vi "CSM Example - State Machine Steps Executed on Sub-Module.vi"() -> ()   [LabVIEW 2017]
doc: "------------- lvcsm -------------\n[CSMStates]\nItem 0 = \"Event Structure\"\nItem 1 = \"Idle\"\nItem 2 = \"CSM Documentation\"\nItem 3 = \"VI Reference\"\nItem 4 = \"Error Handler\"\nItem 5 = \"Critical Error\"\nItem 6 = \"Target Timeout Error\"\nItem 7 = \"Target Error\"\nItem 8 = \"Async Response\"\nItem 9 = \"Response\"\nItem 10 = \"Async Message Posted\"\nItem 11 = \"Initialize Core Data\"\nItem 12 = \"Exit\"\nItem 13 = \"Data: Initialize\"\nItem 14 = \"Data: Cleanup\"\nItem 15 = \"Events: Register\"\nItem 16 = \"Events: Unregister\"\nItem 17 = \"UI: Initialize\"\nItem 18 = \"UI: Cursor Set\"\nItem 19 = \"UI: Front Panel State\"\nItem 20 = \"Macro: Initialize\"\nItem 21 = \"Macro: Exit\"\nItem 22 = \"Macro: SM\"\nItem 23 = \"SM: Step1\"\nItem 24 = \"SM: Step3\"\nItem 25 = \"SM: Event Check\"\n\n[CSMStatus]"
uses:
  user.lib/_NEVSTOP/Communicable State Machine(CSM)/Communicable State Machine.lvlib
panel:
  in  "Exit":bool
  in  "Run":bool
  out "State History of Sub-Module":string
  out "State History of Main":string
  # "SM: Step1\nSM: Step2 @ Sub-Module\nSM: Step3\nSM: Step4 @ Sub-Module\nSM: Event Check"
  # "(back to step1)"
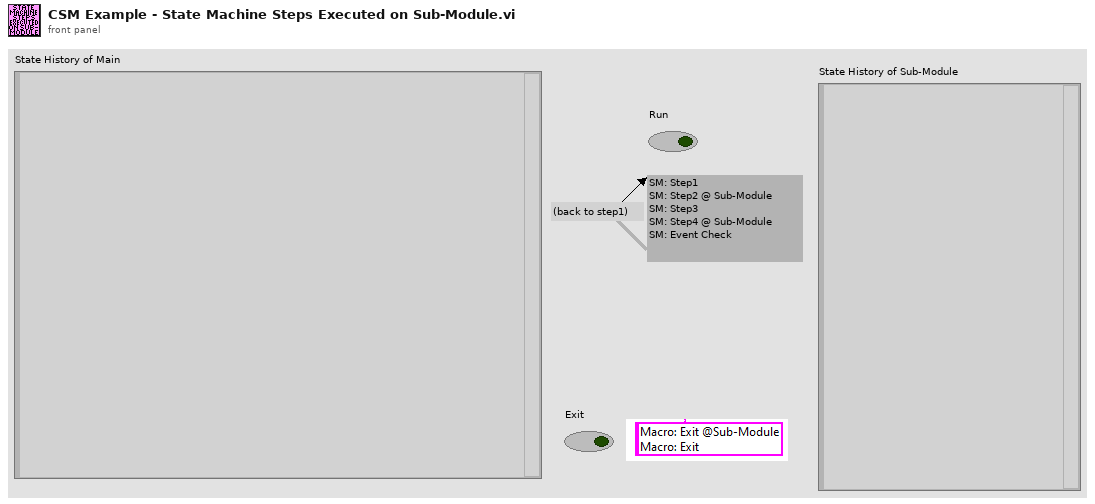
[diagram p1: front panel]
types:
  T1 = enum32{"Invalid", "Standard", "Closed", "Hidden", "Minimized", "Maximized"}
  T2 = enum32{"invalid app kind", "Development System", "Run Time System", "Student Edition", "Embedded LabVIEW", "Evaluation", "Custom"}
  T3 = typedef "Communicable State Machine.lvlib/_CSM_Response Source Message.ctl" = cluster{"‘State":string, "’Arguments":string, "’Error":errorcluster}
  T4 = cluster{"Current VI Reference":refnum<vi>, "Close Panel on Exit?":bool}
  T5 = cluster{"Core":cluster{"Current VI Reference":refnum<vi>, "Close Panel on Exit?":bool}, "Your Boolean data":bool, "State":string}
  T6 = cluster{"Core":cluster{"Current VI Reference":refnum<vi>, "Close Panel on Exit?":bool}, "Your Boolean data":bool, "Your string data":string}
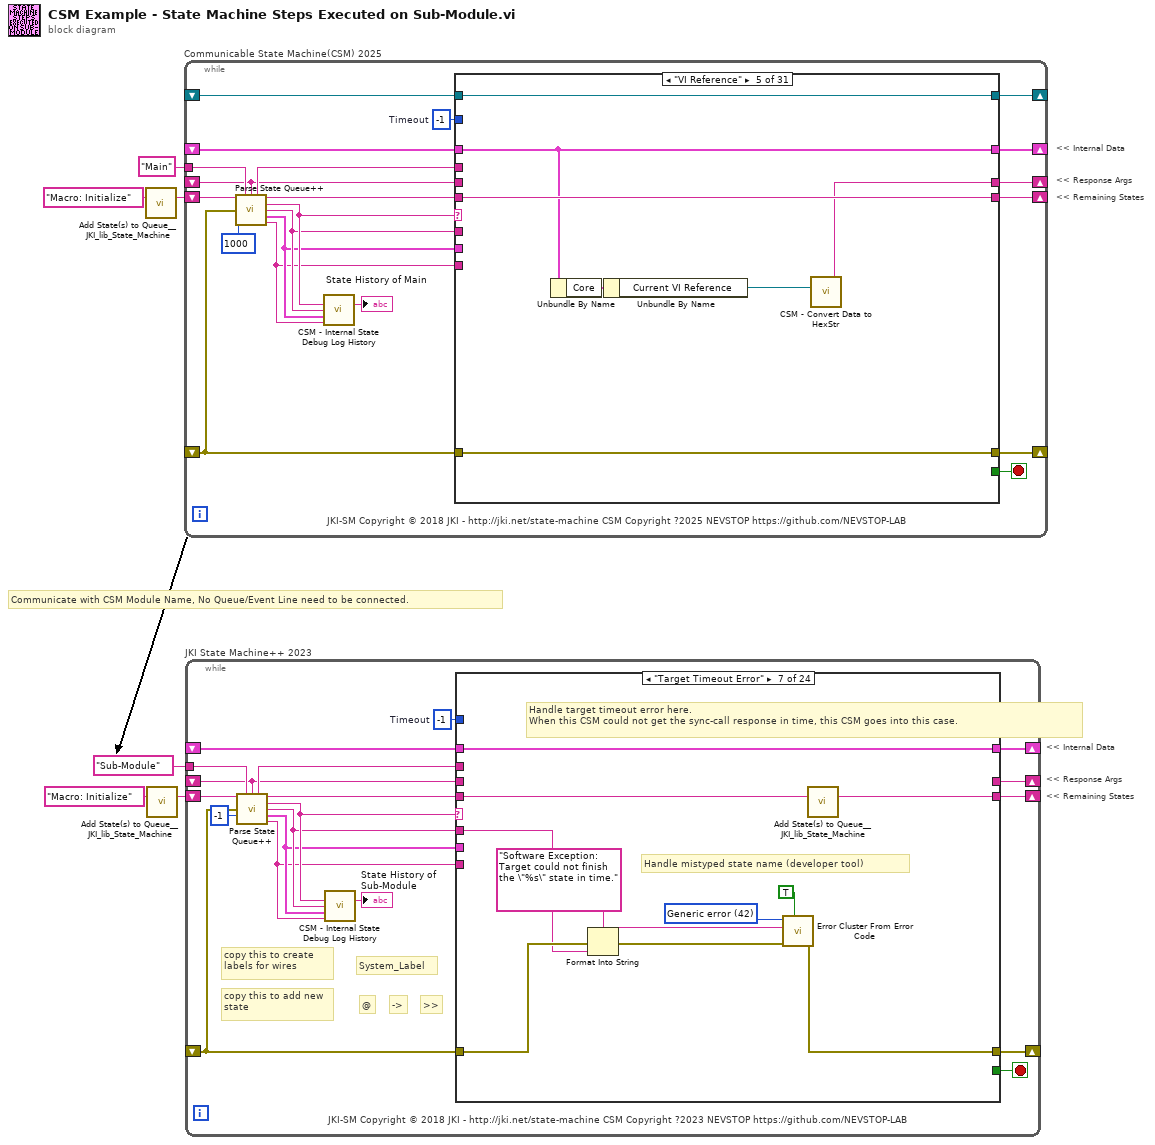
[diagram p0: block diagram]
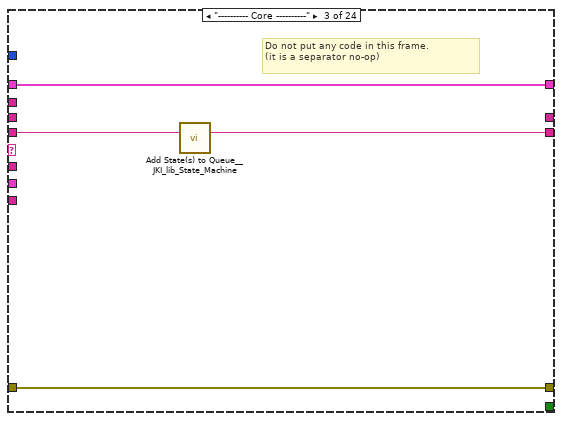
[diagram p4: hidden frame]
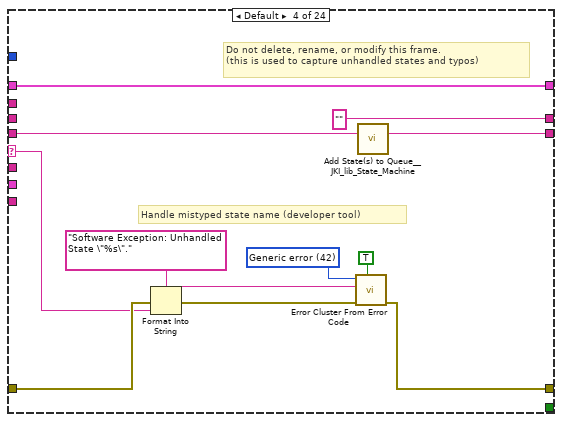
[diagram p5: hidden frame]
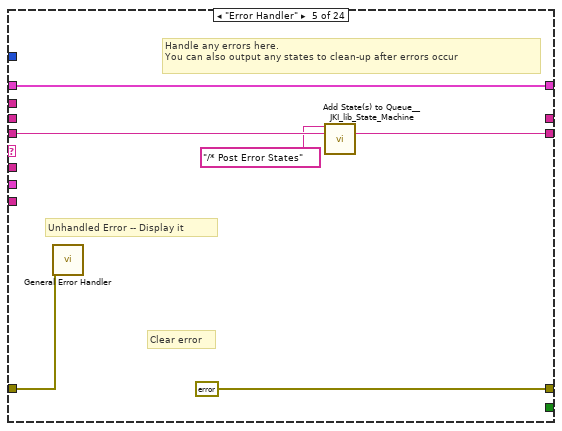
[diagram p6: hidden frame]
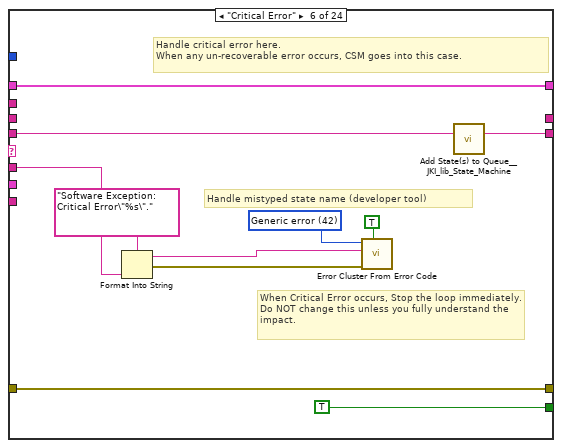
[diagram p7: hidden frame]
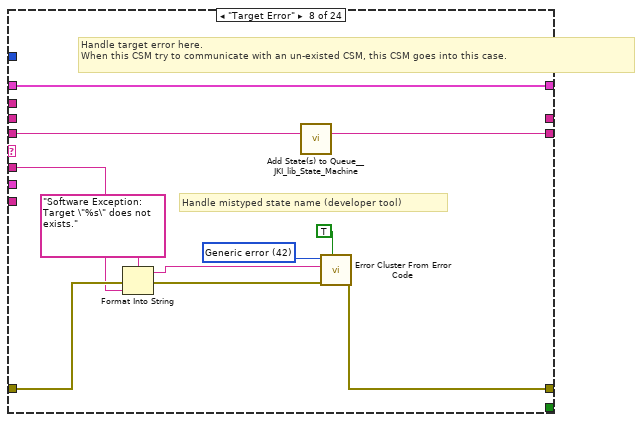
[diagram p8: hidden frame]
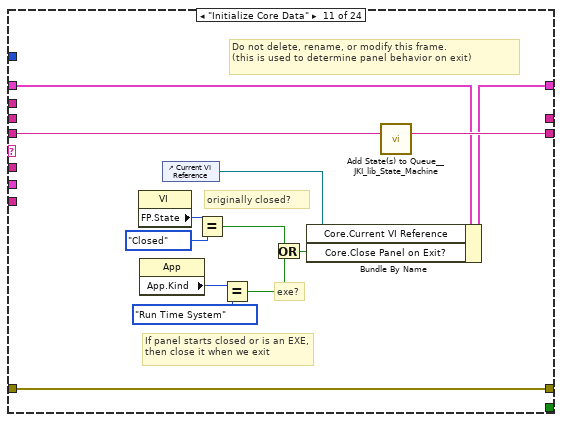
[diagram p11: hidden frame]
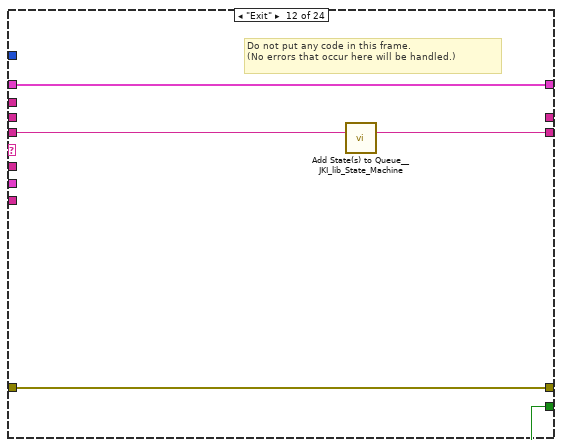
[diagram p12: hidden frame]
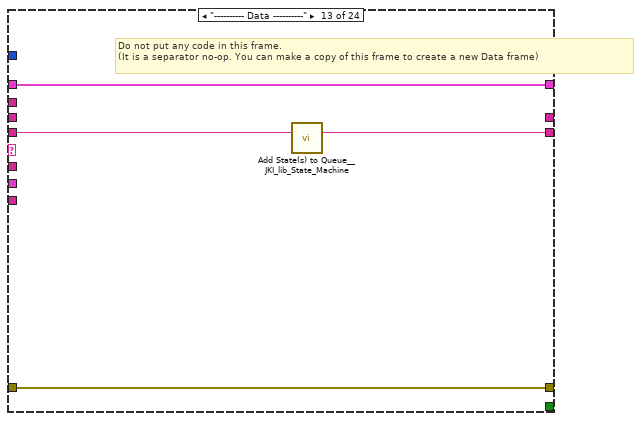
[diagram p13: hidden frame]
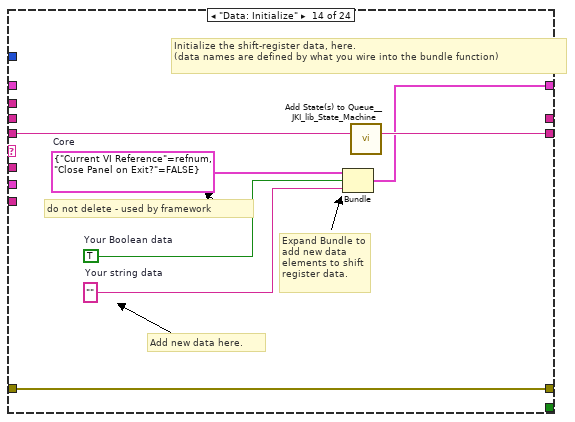
[diagram p14: hidden frame]
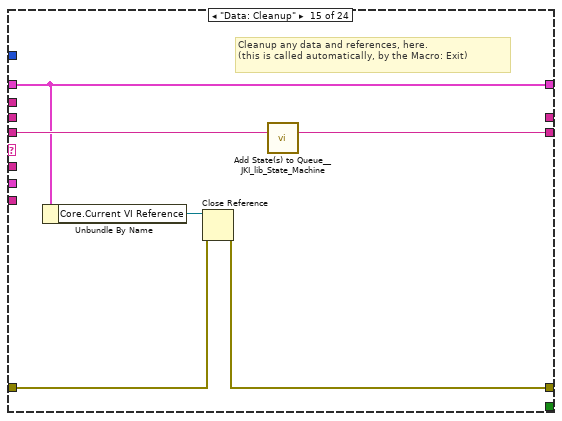
[diagram p15: hidden frame]
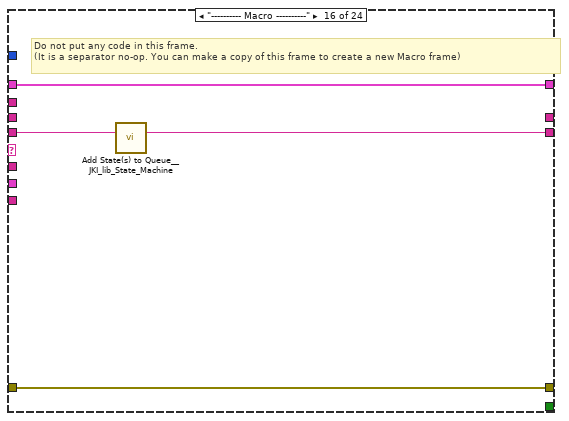
[diagram p16: hidden frame]
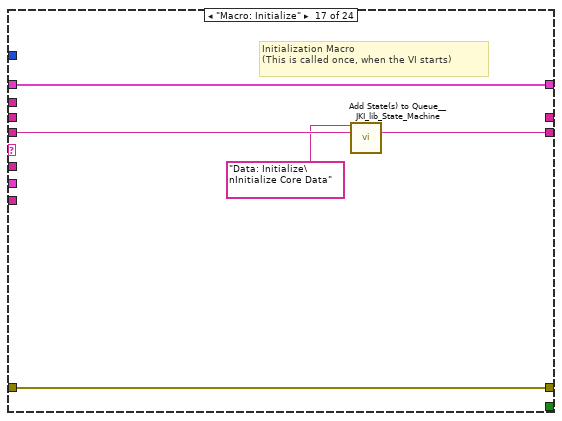
[diagram p17: hidden frame]
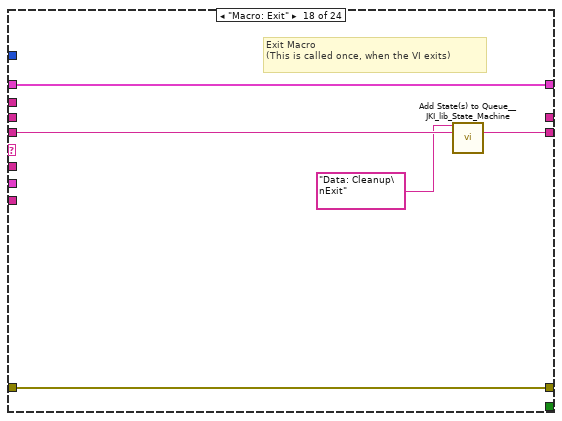
[diagram p18: hidden frame]
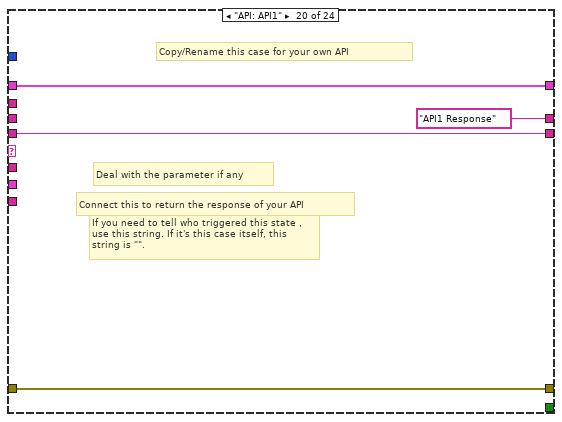
[diagram p20: hidden frame]
diagram:
  # "Communicate with CSM Module Name, No Queue/Event Line need to be connected."
  # "<< Internal Data"
  # "<< Response Args"
  # "<< Remaining States"
  # "<< Internal Data"
  # "<< Response Args"
  # "<< Remaining States"
  n1 = call <vilib>:"Add State(s) to Queue__JKI_lib_State_Machine.vi"("State(s) in (\"\")"="Macro: Initialize") -> ("States Out"=w6:string)  [unwired: 14 in]
  n2 = call <vilib>:"Add State(s) to Queue__JKI_lib_State_Machine.vi"("State(s) in (\"\")"="Macro: Initialize") -> ("States Out"=w1:string)  [unwired: 14 in]
  n3 = while "Communicable State Machine(CSM) 2025" {
    shift-right: [w8] -> _
    shift-left: _ -> [w22]
    shift-right: [w25] -> _
    shift-left: _ -> [w20]
    shift-right: [w24] -> _
    shift-left: w6 -> [w26]
    tunnel: "Main" ("Name(\"\" to use uuid)") -> [w15]
    shift-right: [w18] -> _
    shift-left: _ -> [w9]
    shift-right: [w17] -> _
    shift-left: _ -> [w16]
    stop <- w23 stop-if-true
    w21 = -1  # Timeout
    # "JKI-SM Copyright © 2018 JKI - http://jki.net/state-machine CSM Copyright ?2025 NEVSTOP https://github.com/NEVSTOP-LAB"
    n4 = call "Parse State Queue++.vi"("State Queue"=w26, "Name (\"\" to Use UUID)"=w15, "Response Arguments"=w9, "Previous Error"=w20, "Response Timeout (-2 Use Global Settings)"=1000 ("Response Timeout(1000ms)")) -> ("Name Used"=w10:string, "Remaining States"=w27:string, "Current State"=w14:string, "Arguments"=w13:string, ">> Response Source Message >>"=w12:T3, ">> Source CSM >>"=w11:string)  [unwired: 5 in]
    n5 = call "CSM - Internal State Debug Log History.vi"("State"=w14, "Arguments (\"\")"=w13, ">> Response Source Message >>"=w12, "Source (\"\")"=w11) -> ("Debug Log"=→"State History of Main":string)  [unwired: 11 in]
    n6 = case shown="\"VI Reference\"" w14 {
      selector: w14 -> [_ _ _ w72 _ _ _ _ _ _ _ _ _ _ _ _ _ _ _ _ _ _ _ _ _ _ _ _ _ _ _]
      tunnel: w27 -> [w30 w63 w69 w76 w88 w96 w106 w114 w126 w135 w139 w154 w160 w165 w173 w180 w185 w191 w195 w201 w207 w214 w226 w296 w302 w313 w316 w322 w328 w334 w342]
      tunnel: w13 -> [_ _ _ _ _ _ w99 w110 w122 _ _ _ _ _ _ _ _ _ _ _ _ w209 w220 _ _ _ _ _ _ _ _]
      tunnel: w22 -> [w35 w62 w66 w74 w87 w93 w107 w112 w124 w134 w138 w147 w158 w162 _ w175 w182 w190 w194 w198 w205 w212 w222 w293 w299 w310 w318 w321 w327 w333 w344]
      tunnel: [w34 w64 w67 w78 w89 errorcluster {"status"=FALSE, "code"=0, "source"=""} ("error out") w108 w116 w128 w136 w140 w151 w157 w163 w170 w176 w183 w186 w193 w199 w204 w210 w223 w294 w300 w311 w319 w323 w329 w335 w345] -> w25
      tunnel: w20 -> [w33 w64 w67 w77 w89 w92 w108 w115 w127 w136 w140 w151 w157 w163 w170 w177 w183 _ w196 w199 w204 w211 w224 w294 w300 w311 w319 w323 w329 w335 w345]
      tunnel: [w36 w63 w68 w75 w88 w95 w105 w113 w125 w135 w139 w153 w159 w164 w172 w179 w184 w191 w195 w200 w206 w213 w225 w295 w301 w312 w315 w322 w328 w334 w341] -> w24
      tunnel: [_ _ _ _ _ _ TRUE _ _ _ _ _ TRUE _ _ _ _ _ _ _ _ _ _ _ _ _ _ _ _ _ _] -> w23
      tunnel: [w32 w62 w66 w74 w87 w93 w107 w112 w124 w134 w138 w152 w158 w162 w171 w175 w182 w190 w194 w198 w205 w212 w222 w293 w299 w310 w318 w321 w327 w333 w344] -> w8
      tunnel: w21 -> [w29 _ _ _ _ _ _ _ _ _ _ _ _ _ _ _ _ _ _ _ _ _ _ _ _ _ _ _ _ _ _]
      tunnel: w11 -> [_ _ _ _ _ _ _ _ _ _ _ _ _ _ _ _ _ _ _ _ _ _ _ _ _ _ _ _ _ _ _]
      tunnel: w12 -> [_ _ _ _ _ _ _ _ _ _ _ _ _ _ _ _ _ _ _ _ _ _ _ _ _ _ _ _ _ _ _]
      tunnel: [_ _ _ "" w83 _ _ _ _ _ _ _ _ _ _ _ _ _ _ _ _ _ _ _ _ _ _ _ "Step1 Finished" "Step3 Finished" _] -> w18
      tunnel: [w31 w61 w65 w70 w86 w90 w97 w109 w121 w133 w137 w141 w155 w161 w166 w174 w181 w189 w192 w197 w203 w208 w219 w292 w297 w303 w317 w320 w326 w332 w343] -> w17
      tunnel: w16 -> [w31 w61 w65 w70 w86 w90 w97 w109 w121 w133 w137 w141 w155 w161 w166 w174 w181 _ w192 w197 w203 w208 w219 w292 w297 w303 w317 w320 w326 w332 w343]
      tunnel: w10 -> [_ _ _ _ _ _ _ _ _ _ _ _ _ _ _ _ _ w188 _ _ _ _ _ _ _ _ _ _ _ _ _]
      tunnel: w9 -> [_ _ _ _ _ _ _ _ _ _ _ _ _ _ _ _ _ _ _ _ _ _ _ _ _ _ _ _ _ _ _]
      frame "", "Event Structure", "Idle" {
        # "executes when the state queue is empty"
        n7 = call "Timeout Selector.vi"("Remaining States"=w30, "Timeout Expected"=w29) -> ("Timeout"=w28:i32)  [unwired: 5 in]
        n8 = event shown="[2] \"Run\": Value Change" {
          selector: w31 -> [_ _ _ _ _]
          dyn-events: _ -> [_ _ _ _ _]
          timeout: w28 -> [_ _ _ _ _]
          tunnel: w30 -> [w40 w42 w46 w55 w60]
          tunnel: [w39 w42 w47 w54 w59] -> w36
          tunnel: w35 -> [w37 w43 w48 w52 w57]
          tunnel: [w38 w41 w49 w53 w58] -> w34
          tunnel: w33 -> [w38 w41 w49 w53 w58]
          tunnel: [w37 w43 w48 w52 w57] -> w32
          event Timeout {
            n9 = event-data() -> ()  [unwired: 1 in, 1 out]
            n10 = call <vilib>:"Add State(s) to Queue__JKI_lib_State_Machine.vi"("State(s) in (\"\")"=w40) -> ("States Out"=w39:string)  [unwired: 14 in]
          }
          event User Event {
            # "This user event is used to break out CSM from waiting in the event structure, to process the next state from external. DO NOT place any code here unless you really need to."
            n11 = event-data() -> ()  [unwired: 1 in, 1 out]
          }
          event "Run": Value Change {
            n12 = event-data() -> ("NewVal"=w45:bool)  [unwired: 1 in]
            n13 = call "Add State(s) to Queue By BOOL(Element).vi"("TRUE (\"\")"="Macro: SM" ("TRUE(Empty)"), "Condition"=w45, "State Queue (\"\")"=w46) -> ("Remaining States"=w47:string)  [unwired: 8 in]
          }
          event Panel Close? {
            # "Discard the event because we'll close the front panel ourselves in Macro: Exit"
            # "Close Panel button (pressed) Event\n(this executes Macro: Exit to terminate the VI)"
            n14 = event-data() -> ()  [unwired: 1 in, 1 out]
            n15 = call <vilib>:"Add State(s) to Queue__JKI_lib_State_Machine.vi"("State(s) in Front (\"\")"="Macro: Exit @ Message Handler\nMacro: Exit", "State(s) in (\"\")"=w55) -> ("States Out"=w54:string)  [unwired: 13 in]
            n16 = event-data("Discard?"=TRUE) -> ()  [unwired: 1 in, 1 out]
          }
          event "Exit": Value Change {
            # "Close Panel button (pressed) Event\n(this executes Macro: Exit to terminate the VI)"
            n17 = event-data() -> ()  [unwired: 1 in, 6 out]
            n18 = call <vilib>:"Add State(s) to Queue__JKI_lib_State_Machine.vi"("State(s) in Front (\"\")"="Macro: Exit -@Sub-Module\nMacro: Exit", "State(s) in (\"\")"=w60) -> ("States Out"=w59:string)  [unwired: 13 in]
          }
        }
      }
      frame "CSM Documentation" {
        # "Commenting:\nTo add a comment use \"//\" or \"#\" and all text to the right will be ignored\nCommenting Example:\nUI: Initialize // This initializes the UI\n# This whole line is a comment\n// Another comment line"
        # "State Syntax:\nStateCategory: State >> Argument @ CSMName\nStateCategory: State >> Argument -> CSMName\n\nLine Terminator: Line feed"
        # "CSM Documentation"
      }
      frame "---------- Core ----------" {
        # "Do not put any code in this frame.\n(it is a separator no-op)"
        n19 = call <vilib>:"Add State(s) to Queue__JKI_lib_State_Machine.vi"("State(s) in (\"\")"=w69) -> ("States Out"=w68:string)  [unwired: 14 in]
      }
      frame Default {
        w81 = 42 items=["No error", "Argument error", "Memory is full", "Out of zone", "End of file", "File already open", "Generic file I/O error", "File not found", "File permission error", "Disk is full", "Duplicate path", "Too many files open", "System feature not enabled", "Resource file not found", "Cannot add resource", "Resource not found", "Image not found", "Image memory error", "Pen does not exist", "Config type invalid", "Config token not found", "Config parse error", "Config memory error", "Bad external code format", "Bad external code offset", "External code not present", "Null window", "Destroy window error", "Null menu", "Print aborted", "Bad print record", "Print driver error", "Windows error during printing", "Memory error during printing", "Print dialog error", "Generic print error", "Invalid device refnum", "Device not found", "Device parameter error", "Device unit error", "Cannot open device", "Device call aborted", "Generic error", "Cancelled by user", "Object ID too low", "Object ID too high", "Object not in heap", "Unknown heap", "Unknown object (invalid DefProc)", "Unknown object (DefProc not in table)", "Message out of range", "Invalid (null) method", "Unknown message", "Manager call not supported", "Bad address", "Network operation in progress", "Network operation timed out", "Connection is busy", "Network attribute not supported", "Network error", "Address in use", "System out of memory", "Connection aborted", "Connection refused", "Not connected", "Already connected", "Connection closed", "Initialization error (interapplication manager)", "Bad occurrence", "Wait on unbound occurrence handler", "Occurrence queue overflow", "Datalog type conflict", "Unused", "Unrecognized type (interapplication manager)", "Memory corrupt", "Failed to make temporary DLL", "Old CIN version", "Drag socket not found", "Failed to load drop-object", "Failed to register OLE object", "Failed to release OLE object", "Format specifier type mismatch", "Unknown format specifier", "Too few format specifiers", "Too many format specifiers", "Scan failed", "Newer CIN version", "Error converting to variant", "Runtime menu error", "Password tampered", "Variant attribute not found", "Incompatible variant data type", "Event data is not available", "Event Store is not present", "Occurrence is not found", "Event Queue is not created", "Event info is not available", "Refnum passed is NULL", "Error retrieving Class GUID", "Error retrieving CoClass GUID", "Error retrieving TypeLib GUID.", "Bad built application magic bytes.", "Specific driver is different from the specific driver associated with the Logical Name.", "There is no session opened to the class driver.", "Max Error", "MAX - Error with config objects", "MAX - Error loading configuration", "MAX - Group not supported"]
        # "Do not delete, rename, or modify this frame.\n(this is used to capture unhandled states and typos)"
        # "Handle mistyped state name (developer tool)"
        n20 = Format Into String(format string="Software Exception: Unhandled State \"%s\"." ("message"), error in=w77, w72) -> (resulting string=w80:string, error out=w79:errorcluster)  [unwired: 1 in]
        n21 = call <vilib>:"Error Cluster From Error Code.vi"("show call chain? (False)"=TRUE, "error in (no error)"=w79, "error message (\"\")"=w80, "error code (0)"=w81) -> ("error out"=w78:errorcluster)  [unwired: 5 in]
        n22 = call <vilib>:"Add State(s) to Queue__JKI_lib_State_Machine.vi"("State(s) in (\"\")"=w76) -> ("States Out"=w75:string)  [unwired: 14 in]
      }
      frame "VI Reference" {
        n23 = Unbundle By Name(w87) -> ("Core"=w85:T4)
        n24 = Unbundle By Name(w85) -> ("Current VI Reference"=w84:refnum<vi>)
        n25 = call "CSM - Convert Data to HexStr.vi"("Variant"=w84) -> ("HEX String (0-9,A-F)"=w83:string)  [unwired: 8 in]
      }
      frame "Error Handler" {
        # "Unhandled Error -- Display it"
        # "Handle any errors here.\nYou can also output any states to clean-up after errors occur"
        # "Clear error"
        n26 = call <vilib>:"General Error Handler.vi"("error in (no error)"=w92) -> ()  [unwired: 10 in, 5 out]
        n27 = call <vilib>:"Add State(s) to Queue__JKI_lib_State_Machine.vi"("State(s) in Front (\"\")"="/* Post Error States", "State(s) in (\"\")"=w96) -> ("States Out"=w95:string)  [unwired: 13 in]
      }
      frame "Critical Error" {
        w103 = 42 items=["No error", "Argument error", "Memory is full", "Out of zone", "End of file", "File already open", "Generic file I/O error", "File not found", "File permission error", "Disk is full", "Duplicate path", "Too many files open", "System feature not enabled", "Resource file not found", "Cannot add resource", "Resource not found", "Image not found", "Image memory error", "Pen does not exist", "Config type invalid", "Config token not found", "Config parse error", "Config memory error", "Bad external code format", "Bad external code offset", "External code not present", "Null window", "Destroy window error", "Null menu", "Print aborted", "Bad print record", "Print driver error", "Windows error during printing", "Memory error during printing", "Print dialog error", "Generic print error", "Invalid device refnum", "Device not found", "Device parameter error", "Device unit error", "Cannot open device", "Device call aborted", "Generic error", "Cancelled by user", "Object ID too low", "Object ID too high", "Object not in heap", "Unknown heap", "Unknown object (invalid DefProc)", "Unknown object (DefProc not in table)", "Message out of range", "Invalid (null) method", "Unknown message", "Manager call not supported", "Bad address", "Network operation in progress", "Network operation timed out", "Connection is busy", "Network attribute not supported", "Network error", "Address in use", "System out of memory", "Connection aborted", "Connection refused", "Not connected", "Already connected", "Connection closed", "Initialization error (interapplication manager)", "Bad occurrence", "Wait on unbound occurrence handler", "Occurrence queue overflow", "Datalog type conflict", "Unused", "Unrecognized type (interapplication manager)", "Memory corrupt", "Failed to make temporary DLL", "Old CIN version", "Drag socket not found", "Failed to load drop-object", "Failed to register OLE object", "Failed to release OLE object", "Format specifier type mismatch", "Unknown format specifier", "Too few format specifiers", "Too many format specifiers", "Scan failed", "Newer CIN version", "Error converting to variant", "Runtime menu error", "Password tampered", "Variant attribute not found", "Incompatible variant data type", "Event data is not available", "Event Store is not present", "Occurrence is not found", "Event Queue is not created", "Event info is not available", "Refnum passed is NULL", "Error retrieving Class GUID", "Error retrieving CoClass GUID", "Error retrieving TypeLib GUID.", "Bad built application magic bytes.", "Specific driver is different from the specific driver associated with the Logical Name.", "There is no session opened to the class driver.", "Max Error", "MAX - Error with config objects", "MAX - Error loading configuration", "MAX - Group not supported"]
        # "Handle critical error here.\nWhen any un-recoverable error occurs, CSM goes into this case."
        # "When Critical Error occurs, Stop the loop immediately. Do NOT change this unless you fully understand the impact."
        # "Handle mistyped state name (developer tool)"
        n28 = Format Into String(format string="Software Exception: Critical Error\"%s\"." ("message"), w99) -> (resulting string=w102:string, error out=w101:errorcluster)  [unwired: 2 in]
        n29 = call <vilib>:"Error Cluster From Error Code.vi"("show call chain? (False)"=TRUE, "error in (no error)"=w101, "error message (\"\")"=w102, "error code (0)"=w103) -> ()  [unwired: 5 in, 1 out]
        n30 = call <vilib>:"Add State(s) to Queue__JKI_lib_State_Machine.vi"("State(s) in (\"\")"=w106) -> ("States Out"=w105:string)  [unwired: 14 in]
      }
      frame "Target Timeout Error" {
        w119 = 42 items=["No error", "Argument error", "Memory is full", "Out of zone", "End of file", "File already open", "Generic file I/O error", "File not found", "File permission error", "Disk is full", "Duplicate path", "Too many files open", "System feature not enabled", "Resource file not found", "Cannot add resource", "Resource not found", "Image not found", "Image memory error", "Pen does not exist", "Config type invalid", "Config token not found", "Config parse error", "Config memory error", "Bad external code format", "Bad external code offset", "External code not present", "Null window", "Destroy window error", "Null menu", "Print aborted", "Bad print record", "Print driver error", "Windows error during printing", "Memory error during printing", "Print dialog error", "Generic print error", "Invalid device refnum", "Device not found", "Device parameter error", "Device unit error", "Cannot open device", "Device call aborted", "Generic error", "Cancelled by user", "Object ID too low", "Object ID too high", "Object not in heap", "Unknown heap", "Unknown object (invalid DefProc)", "Unknown object (DefProc not in table)", "Message out of range", "Invalid (null) method", "Unknown message", "Manager call not supported", "Bad address", "Network operation in progress", "Network operation timed out", "Connection is busy", "Network attribute not supported", "Network error", "Address in use", "System out of memory", "Connection aborted", "Connection refused", "Not connected", "Already connected", "Connection closed", "Initialization error (interapplication manager)", "Bad occurrence", "Wait on unbound occurrence handler", "Occurrence queue overflow", "Datalog type conflict", "Unused", "Unrecognized type (interapplication manager)", "Memory corrupt", "Failed to make temporary DLL", "Old CIN version", "Drag socket not found", "Failed to load drop-object", "Failed to register OLE object", "Failed to release OLE object", "Format specifier type mismatch", "Unknown format specifier", "Too few format specifiers", "Too many format specifiers", "Scan failed", "Newer CIN version", "Error converting to variant", "Runtime menu error", "Password tampered", "Variant attribute not found", "Incompatible variant data type", "Event data is not available", "Event Store is not present", "Occurrence is not found", "Event Queue is not created", "Event info is not available", "Refnum passed is NULL", "Error retrieving Class GUID", "Error retrieving CoClass GUID", "Error retrieving TypeLib GUID.", "Bad built application magic bytes.", "Specific driver is different from the specific driver associated with the Logical Name.", "There is no session opened to the class driver.", "Max Error", "MAX - Error with config objects", "MAX - Error loading configuration", "MAX - Group not supported"]
        # "Handle target timeout error here.\nWhen this CSM could not get the sync-call response in time, this CSM goes into this case."
        # "Handle mistyped state name (developer tool)"
        n31 = Format Into String(format string="Software Exception: Target could not finish the \"%s\" state in time." ("message"), error in=w115, w110) -> (resulting string=w118:string, error out=w117:errorcluster)  [unwired: 1 in]
        n32 = call <vilib>:"Error Cluster From Error Code.vi"("show call chain? (False)"=TRUE, "error in (no error)"=w117, "error message (\"\")"=w118, "error code (0)"=w119) -> ("error out"=w116:errorcluster)  [unwired: 5 in]
        n33 = call <vilib>:"Add State(s) to Queue__JKI_lib_State_Machine.vi"("State(s) in (\"\")"=w114) -> ("States Out"=w113:string)  [unwired: 14 in]
      }
      frame "Target Error" {
        w131 = 42 items=["No error", "Argument error", "Memory is full", "Out of zone", "End of file", "File already open", "Generic file I/O error", "File not found", "File permission error", "Disk is full", "Duplicate path", "Too many files open", "System feature not enabled", "Resource file not found", "Cannot add resource", "Resource not found", "Image not found", "Image memory error", "Pen does not exist", "Config type invalid", "Config token not found", "Config parse error", "Config memory error", "Bad external code format", "Bad external code offset", "External code not present", "Null window", "Destroy window error", "Null menu", "Print aborted", "Bad print record", "Print driver error", "Windows error during printing", "Memory error during printing", "Print dialog error", "Generic print error", "Invalid device refnum", "Device not found", "Device parameter error", "Device unit error", "Cannot open device", "Device call aborted", "Generic error", "Cancelled by user", "Object ID too low", "Object ID too high", "Object not in heap", "Unknown heap", "Unknown object (invalid DefProc)", "Unknown object (DefProc not in table)", "Message out of range", "Invalid (null) method", "Unknown message", "Manager call not supported", "Bad address", "Network operation in progress", "Network operation timed out", "Connection is busy", "Network attribute not supported", "Network error", "Address in use", "System out of memory", "Connection aborted", "Connection refused", "Not connected", "Already connected", "Connection closed", "Initialization error (interapplication manager)", "Bad occurrence", "Wait on unbound occurrence handler", "Occurrence queue overflow", "Datalog type conflict", "Unused", "Unrecognized type (interapplication manager)", "Memory corrupt", "Failed to make temporary DLL", "Old CIN version", "Drag socket not found", "Failed to load drop-object", "Failed to register OLE object", "Failed to release OLE object", "Format specifier type mismatch", "Unknown format specifier", "Too few format specifiers", "Too many format specifiers", "Scan failed", "Newer CIN version", "Error converting to variant", "Runtime menu error", "Password tampered", "Variant attribute not found", "Incompatible variant data type", "Event data is not available", "Event Store is not present", "Occurrence is not found", "Event Queue is not created", "Event info is not available", "Refnum passed is NULL", "Error retrieving Class GUID", "Error retrieving CoClass GUID", "Error retrieving TypeLib GUID.", "Bad built application magic bytes.", "Specific driver is different from the specific driver associated with the Logical Name.", "There is no session opened to the class driver.", "Max Error", "MAX - Error with config objects", "MAX - Error loading configuration", "MAX - Group not supported"]
        # "Handle target error here.\nWhen this CSM try to communicate with an un-existed CSM, this CSM goes into this case."
        # "Handle mistyped state name (developer tool)"
        n34 = Format Into String(format string="Software Exception: Target \"%s\" does not exists." ("message"), error in=w127, w122) -> (resulting string=w130:string, error out=w129:errorcluster)  [unwired: 1 in]
        n35 = call <vilib>:"Add State(s) to Queue__JKI_lib_State_Machine.vi"("State(s) in (\"\")"=w126) -> ("States Out"=w125:string)  [unwired: 14 in]
        n36 = call <vilib>:"Error Cluster From Error Code.vi"("show call chain? (False)"=TRUE, "error in (no error)"=w129, "error message (\"\")"=w130, "error code (0)"=w131) -> ("error out"=w128:errorcluster)  [unwired: 5 in]
      }
      frame "Async Response", "Response" {
        # "Handle Async-call Response (\"Async Response\" for ->)"
        # "Handle Sync-call Response (\"Response\" for @)"
        # "After Message is executed, CSM goes to this state for receive the response. \n    For Async Message(->), \"Async Response\" is used. This CSM will goes to \"Async Message Posted\" immediately and receive the \"Async Response\" after the callee finishes the message.\n    For Sync Message(@),  This CSM will wait until the message is done and immediately goes to \"Response\""
      }
      frame "Async Message Posted" {
        # "Handle post action for async message (->)."
        # "After Async Message is posted (->), CSM goes to this state for post-action. You can use Argument - State to tell which Async Message is called."
      }
      frame "Initialize Core Data" {
        # "Do not delete, rename, or modify this frame.\n(this is used to determine panel behavior on exit)"
        # "originally closed?"
        # "exe?"
        # "If panel starts closed or is an EXE, then close it when we exit"
        n37 = property class="VI"() -> ("FP.State"=w144:T1)  [unwired: 2 in, 2 out]
        n38 = property class="App"() -> ("App.Kind"=w150:T2)  [unwired: 2 in, 2 out]
        n39 = control-ref of="Current VI Reference"() -> (w145:refnum<vi>)
        n40 = Equal?(x=w144, y=T1."Closed" ("Front Panel Window:State")) -> (x = y?=w142:bool)
        n41 = Equal?(x=w150, y=T2."Run Time System" ("Application:Kind")) -> (x = y?=w148:bool)
        n42 = Or(x=w142, y=w148) -> (x .or. y?=w146:bool)
        n43 = Bundle By Name(cluster=w147, "Core.Current VI Reference"=w145, "Core.Close Panel on Exit?"=w146) -> (w152:T5)
        n44 = call <vilib>:"Add State(s) to Queue__JKI_lib_State_Machine.vi"("State(s) in (\"\")"=w154) -> ("States Out"=w153:string)  [unwired: 14 in]
      }
      frame "Exit" {
        # "Do not put any code in this frame.\n(No errors that occur here will be handled.)"
        n45 = call <vilib>:"Add State(s) to Queue__JKI_lib_State_Machine.vi"("State(s) in (\"\")"=w160) -> ("States Out"=w159:string)  [unwired: 14 in]
      }
      frame "---------- Data ----------" {
        # "Do not put any code in this frame.\n(It is a separator no-op. You can make a copy of this frame to create a new Data frame)"
        n46 = call <vilib>:"Add State(s) to Queue__JKI_lib_State_Machine.vi"("State(s) in (\"\")"=w165) -> ("States Out"=w164:string)  [unwired: 14 in]
      }
      frame "Data: Initialize" {
        w167 = T4 {"Current VI Reference"=refnum, "Close Panel on Exit?"=FALSE}  # Core
        w169 = TRUE  # Your Boolean data
        w168 = ""  # State
        # "do not delete - used by framework"
        # "Initialize the shift-register data, here.\n(data names are defined by what you wire into the bundle function)"
        n47 = Bundle("Core"=w167, "Your Boolean data"=w169, "State"=w168) -> (w171:T5)  [unwired: 1 in]
        n48 = call <vilib>:"Add State(s) to Queue__JKI_lib_State_Machine.vi"("State(s) in (\"\")"=w173) -> ("States Out"=w172:string)  [unwired: 14 in]
      }
      frame "Data: Cleanup" {
        # "Cleanup any data and references, here.\n(this is called automatically, by the Macro: Exit)"
        n49 = Unbundle By Name(w175) -> ("Core.Current VI Reference"=w178:refnum<vi>)
        n50 = Close Reference(reference=w178, error in (no error)=w177) -> (error out=w176:errorcluster)
        n51 = call <vilib>:"Add State(s) to Queue__JKI_lib_State_Machine.vi"("State(s) in (\"\")"=w180) -> ("States Out"=w179:string)  [unwired: 14 in]
      }
      frame "---------- Events ----------" {
        # "Do not put any code in this frame.\n(It is a separator no-op. You can make a copy of this frame to create a new UI frame)"
        n52 = call <vilib>:"Add State(s) to Queue__JKI_lib_State_Machine.vi"("State(s) in (\"\")"=w185) -> ("States Out"=w184:string)  [unwired: 14 in]
      }
      frame "Events: Register" {
        # "Register message event to break Waiting in Event structure."
        n53 = call "CSM - Get New State Notifier Event.vi"("Name (\"\" to Use UUID) In"=w188) -> ("error out"=w186:errorcluster, "New State Notifier Event"=w187:refnum<user-event>)  [unwired: 9 in]
        n54 = register-events(w187) -> (reference out=w189:refnum<event-registration>)  [unwired: 2 in, 1 out]
      }
      frame "Events: Unregister" {
        n55 = Unregister For Events(event registration refnum=w192, error in=w196) -> (error out=w193:errorcluster)
      }
      frame "---------- UI ----------" {
        # "Do not put any code in this frame.\n(It is a separator no-op. You can make a copy of this frame to create a new UI frame)"
        n56 = call <vilib>:"Add State(s) to Queue__JKI_lib_State_Machine.vi"("State(s) in (\"\")"=w201) -> ("States Out"=w200:string)  [unwired: 14 in]
      }
      frame "UI: Initialize" {
        # "Initialize the User Interface, here.\n(this is called automatically, by the Macro: Init)"
        n57 = local write "Run"(FALSE ("Run")) -> ()
        n58 = call <vilib>:"Add State(s) to Queue__JKI_lib_State_Machine.vi"("State(s) in (\"\")"=w207) -> ("States Out"=w206:string)  [unwired: 14 in]
      }
      frame "UI: Cursor Set" {
        # "Argument"
        # "Set and Unset Cursor Busy.\n(Usage: \"UI: Cursor Set >> Busy|Idle\")"
        n59 = case shown="\"Idle\", Default" w209 {
          tunnel: w211 -> [w216 w218]
          tunnel: [w215 w217] -> w210
          frame "Idle", Default {
            n60 = call <vilib>:"Unset Busy.vi"("error in (no error)"=w216) -> ("error out"=w215:errorcluster)  [unwired: 10 in]
          }
          frame "Busy" {
            n61 = call <vilib>:"Set Busy.vi"("error in (no error)"=w218) -> ("error out"=w217:errorcluster)  [unwired: 9 in, 1 out]
          }
        }
        n62 = call <vilib>:"Add State(s) to Queue__JKI_lib_State_Machine.vi"("State(s) in (\"\")"=w214) -> ("States Out"=w213:string)  [unwired: 14 in]
      }
      frame "UI: Front Panel State" {
        # "Argument"
        # "Set Front Panel Open or Closed\n(Usage: \"UI: Front Panel State >> Open|Close\")"
        n63 = Unbundle By Name(w222) -> ("Core.Current VI Reference"=w221:refnum<vi>)
        n64 = call <vilib>:"Add State(s) to Queue__JKI_lib_State_Machine.vi"("State(s) in (\"\")"=w226) -> ("States Out"=w225:string)  [unwired: 14 in]
        n65 = case shown="\"Minimize\", \"Minimized\"" w220 {
          tunnel: w224 -> [w232 w247 w258 w271 w284]
          tunnel: [w234 w248 w260 w273 w286] -> w223
          tunnel: w221 -> [w233 w245 w259 w272 w285]
          frame "Open", "Standard", Default {
            w227 = T1."Standard" ("State")
            n66 = property class="VI"(reference=w233, error in=w232) -> (reference out=w230:refnum<vi>, error out=w231:errorcluster, "FP.State"=w229:T1)
            n67 = Not Equal?(x=w229, y=w227) -> (x != y?=w228:bool)
            n68 = case shown="True" w228 {
              tunnel: [w238 w240] -> w234
              tunnel: w231 -> [w237 w240]
              tunnel: w230 -> [w236 _]
              tunnel: w227 -> [w235 _]
              frame True {
                n69 = invoke class="VI" method="FP.Open"(reference=w236, error in=w237, "Activate"=TRUE, "State"=w235) -> (error out=w238:errorcluster)  [unwired: 1 in, 4 out]
              }
              frame False {
              }
            }
          }
          frame "Close", "Closed" {
            n70 = property class="VI"(reference=w245, error in=w247) -> (reference out=w244:refnum<vi>, error out=w246:errorcluster, "FP.State"=w242:T1)
            n71 = Not Equal?(x=w242, y=T1."Closed" ("Front Panel Window:State")) -> (x != y?=w241:bool)
            n72 = case shown="True" w241 {
              tunnel: [w249 w252] -> w248
              tunnel: w246 -> [w249 w251]
              tunnel: w244 -> [_ w250]
              frame False {
              }
              frame True {
                n73 = invoke class="VI" method="FP.Close"(reference=w250, error in=w251) -> (error out=w252:errorcluster)  [unwired: 1 in, 2 out]
              }
            }
          }
          frame "Hidden", "Hide" {
            w253 = T1."Hidden" ("State")
            n74 = property class="VI"(reference=w259, error in=w258) -> (reference out=w256:refnum<vi>, error out=w257:errorcluster, "FP.State"=w255:T1)
            n75 = Not Equal?(x=w255, y=w253) -> (x != y?=w254:bool)
            n76 = case shown="True" w254 {
              tunnel: [w264 w265] -> w260
              tunnel: w257 -> [w263 w265]
              tunnel: w256 -> [w262 _]
              tunnel: w253 -> [w261 _]
              frame True {
                n77 = invoke class="VI" method="FP.Open"(reference=w262, error in=w263, "State"=w261) -> (error out=w264:errorcluster)  [unwired: 2 in, 4 out]
              }
              frame False {
              }
            }
          }
          frame "Minimize", "Minimized" {
            w266 = T1."Minimized" ("State")
            n78 = property class="VI"(reference=w272, error in=w271) -> (reference out=w269:refnum<vi>, error out=w270:errorcluster, "FP.State"=w268:T1)
            n79 = Not Equal?(x=w268, y=w266) -> (x != y?=w267:bool)
            n80 = case shown="True" w267 {
              tunnel: [w277 w278] -> w273
              tunnel: w270 -> [w276 w278]
              tunnel: w269 -> [w275 _]
              tunnel: w266 -> [w274 _]
              frame True {
                n81 = invoke class="VI" method="FP.Open"(reference=w275, error in=w276, "State"=w274) -> (error out=w277:errorcluster)  [unwired: 2 in, 4 out]
              }
              frame False {
              }
            }
          }
          frame "Maximize", "Maximized" {
            w279 = T1."Maximized" ("State")
            n82 = property class="VI"(reference=w285, error in=w284) -> (reference out=w282:refnum<vi>, error out=w283:errorcluster, "FP.State"=w281:T1)
            n83 = Not Equal?(x=w281, y=w279) -> (x != y?=w280:bool)
            n84 = case shown="True" w280 {
              tunnel: [w290 w291] -> w286
              tunnel: w283 -> [w289 w291]
              tunnel: w282 -> [w288 _]
              tunnel: w279 -> [w287 _]
              frame True {
                n85 = invoke class="VI" method="FP.Open"(reference=w288, error in=w289, "State"=w287) -> (error out=w290:errorcluster)  [unwired: 2 in, 4 out]
              }
              frame False {
              }
            }
          }
        }
      }
      frame "---------- Macro ----------" {
        # "Do not put any code in this frame.\n(It is a separator no-op. You can make a copy of this frame to create a new Macro frame)"
        n86 = call <vilib>:"Add State(s) to Queue__JKI_lib_State_Machine.vi"("State(s) in (\"\")"=w296) -> ("States Out"=w295:string)  [unwired: 14 in]
      }
      frame "Macro: Initialize" {
        w298 = "Data: Initialize\nInitialize Core Data\nEvents: Register\nUI: Initialize\nUI: Front Panel State >> Open"  # Data: Initialize Initialize Core Data Events: Register UI: Initialize UI: Front Panel State >> Open
        # "Initialization Macro\n(This is called once, when the VI starts)"
        n87 = call <vilib>:"Add State(s) to Queue__JKI_lib_State_Machine.vi"("State(s) in Front (\"\")"=w298, "State(s) in (\"\")"=w302) -> ("States Out"=w301:string)  [unwired: 13 in]
      }
      frame "Macro: Exit" {
        # "Exit Macro\n(This is called once, when the VI exits)"
        n88 = Unbundle By Name(w310) -> ("Core.Close Panel on Exit?"=w309:bool)
        n89 = Select(t="UI: Front Panel State >> Close", s=w309, f="") -> (s? t:f=w306:string)
        n90 = call <vilib>:"Add State(s) to Queue__JKI_lib_State_Machine.vi"("State(s) in (\"\")"=w306, "State(s) at Back (\"\")"="Data: Cleanup\nEvents: Unregister\nExit") -> ("States Out"=w304:string)  [unwired: 13 in]
        n91 = call <vilib>:"Add State(s) to Queue__JKI_lib_State_Machine.vi"("State(s) in Front (\"\")"=w304, "State(s) in (\"\")"=w313) -> ("States Out"=w312:string)  [unwired: 13 in]
      }
      frame "Macro: SM" {
        n92 = call <vilib>:"Add State(s) to Queue__JKI_lib_State_Machine.vi"("State(s) in Front (\"\")"="SM: Step1\nSM: Step2 -@ Sub-Module\nSM: Step3\nSM: Step4 -@ Sub-Module\nSM: Event Check" ("State(s) in Front (\"\")"), "State(s) in (\"\")"=w316) -> ("States Out"=w315:string)  [unwired: 13 in]
      }
      frame "---State Machine ---" {
      }
      frame "SM: Step1" {
        n93 = Wait (ms)(milliseconds to wait=u32 500) -> ()  [unwired: 1 out]
      }
      frame "SM: Step3" {
        n94 = Wait (ms)(milliseconds to wait=u32 500) -> ()  [unwired: 1 out]
      }
      frame "SM: Event Check" {
        n95 = Wait (ms)(milliseconds to wait=u32 500) -> ()  [unwired: 1 out]
        n96 = call "Add State(s) to Queue By BOOL(Element).vi"("TRUE (\"\")"="Macro: SM" ("TRUE(Empty)"), "Condition"="Run", "State Queue (\"\")"="Idle" ("State(s) in Front (\"\")")) -> ("Remaining States"=w339:string)  [unwired: 8 in]
        n97 = call <vilib>:"Add State(s) to Queue__JKI_lib_State_Machine.vi"("State(s) in Front (\"\")"=w339, "State(s) in (\"\")"=w342) -> ("States Out"=w341:string)  [unwired: 13 in]
      }
    }
  }
  n98 = while "JKI State Machine++ 2023" {
    shift-right: [w359] -> _
    shift-left: _ -> [w358]
    shift-right: [w362] -> _
    shift-left: _ -> [w356]
    shift-right: [w361] -> _
    shift-left: w1 -> [w363]
    tunnel: "Sub-Module" ("Name(\"\" to use uuid) 2") -> [w354]
    shift-right: [w355] -> _
    shift-left: _ -> [w348]
    stop <- w360 stop-if-true
    w357 = -1  # Timeout
    # "JKI-SM Copyright © 2018 JKI - http://jki.net/state-machine CSM Copyright ?2023 NEVSTOP https://github.com/NEVSTOP-LAB"
    # "copy this to add new state"
    # ">>"
    # "->"
    # "@"
    # "copy this to create labels for wires"
    # "System_Label"
    n99 = call "Parse State Queue++.vi"("State Queue"=w363, "Name (\"\" to Use UUID)"=w354, "Response Arguments"=w348, "Previous Error"=w356, "Dequeue (1 ms)"=-1 ("Dequeue Timeout(0ms)")) -> ("Name Used"=w349:string, "Remaining States"=w364:string, "Current State"=w353:string, "Arguments"=w352:string, ">> Response Source Message >>"=w351:T3, ">> Source CSM >>"=w350:string)  [unwired: 5 in]
    n100 = call "CSM - Internal State Debug Log History.vi"("State"=w353, "Arguments (\"\")"=w352, ">> Response Source Message >>"=w351, "Source (\"\")"=w350) -> ("Debug Log"=→"State History of Sub-Module":string)  [unwired: 11 in]
    n101 = case shown="\"Target Timeout Error\"" w353 {
      selector: w353 -> [_ _ _ w376 _ _ _ _ _ _ _ _ _ _ _ _ _ _ _ _ _ _ _ _]
      tunnel: w364 -> [w366 w369 w374 w380 w392 w401 w408 w419 w427 w430 w444 w449 w453 w460 w466 w470 w475 w480 w482 w486 w491 w498 w504 w510]
      tunnel: w352 -> [_ _ _ _ _ w394 w404 w415 _ _ _ _ _ _ _ _ _ _ _ _ w489 _ _ _]
      tunnel: w358 -> [w367 w368 w371 w378 w389 w402 w406 w417 w426 w429 w437 w447 w450 _ w461 w467 w472 w477 w481 w485 w490 w495 w501 w507]
      tunnel: [w365 w370 w372 w382 errorcluster {"status"=FALSE, "code"=0, "source"=""} ("error out") w403 w410 w421 w428 w431 w441 w446 w451 w457 w462 w468 w473 w478 w483 w487 w492 w496 w502 w508] -> w362
      tunnel: w356 -> [w365 w370 w372 w381 w388 w403 w409 w420 w428 w431 w441 w446 w451 w457 w463 w468 w473 w478 w483 w487 w492 w496 w502 w508]
      tunnel: [w366 w369 w373 w379 w391 w400 w407 w418 w427 w430 w443 w448 w452 w459 w465 w469 w474 w479 w482 w486 w491 w497 w503 w509] -> w361
      tunnel: [_ _ _ _ _ TRUE _ _ _ _ _ TRUE _ _ _ _ _ _ _ _ _ _ _ _] -> w360
      tunnel: [w367 w368 w371 w378 w389 w402 w406 w417 w426 w429 w442 w447 w450 w458 w461 w467 w472 w477 w481 w485 w490 w495 w501 w507] -> w359
      tunnel: w357 -> [_ _ _ _ _ _ _ _ _ _ _ _ _ _ _ _ _ _ _ _ _ _ _ _]
      tunnel: w350 -> [_ _ _ _ _ _ _ _ _ _ _ _ _ _ _ _ _ _ _ _ _ _ _ _]
      tunnel: w351 -> [_ _ _ _ _ _ _ _ _ _ _ _ _ _ _ _ _ _ _ _ _ _ _ _]
      tunnel: [_ _ _ "" _ _ _ _ _ _ _ _ _ _ _ _ _ _ _ "API1 Response" w488 _ "Step2 Finished" "Step4 Finished"] -> w355
      tunnel: w349 -> [_ _ _ _ _ _ _ _ _ _ _ _ _ _ _ _ _ _ _ _ _ _ _ _]
      tunnel: w348 -> [_ _ _ _ _ _ _ _ _ _ _ _ _ _ _ _ _ _ _ _ _ _ _ _]
      frame "", "Idle" {
        # "executes when the state queue is empty"
      }
      frame "CSM Documentation" {
        # "Commenting:\nTo add a comment use \"//\" or \"#\" and all text to the right will be ignored\nCommenting Example:\nUI: Initialize // This initializes the UI\n# This whole line is a comment\n// Another comment line"
        # "State Syntax:\nStateCategory: State >> Argument @ CSMName\nStateCategory: State >> Argument -> CSMName\n\nLine Terminator: Line feed"
        # "CSM Documentation"
      }
      frame "---------- Core ----------" {
        # "Do not put any code in this frame.\n(it is a separator no-op)"
        n102 = call <vilib>:"Add State(s) to Queue__JKI_lib_State_Machine.vi"("State(s) in (\"\")"=w374) -> ("States Out"=w373:string)  [unwired: 14 in]
      }
      frame Default {
        w385 = 42 items=["No error", "Argument error", "Memory is full", "Out of zone", "End of file", "File already open", "Generic file I/O error", "File not found", "File permission error", "Disk is full", "Duplicate path", "Too many files open", "System feature not enabled", "Resource file not found", "Cannot add resource", "Resource not found", "Image not found", "Image memory error", "Pen does not exist", "Config type invalid", "Config token not found", "Config parse error", "Config memory error", "Bad external code format", "Bad external code offset", "External code not present", "Null window", "Destroy window error", "Null menu", "Print aborted", "Bad print record", "Print driver error", "Windows error during printing", "Memory error during printing", "Print dialog error", "Generic print error", "Invalid device refnum", "Device not found", "Device parameter error", "Device unit error", "Cannot open device", "Device call aborted", "Generic error", "Cancelled by user", "Object ID too low", "Object ID too high", "Object not in heap", "Unknown heap", "Unknown object (invalid DefProc)", "Unknown object (DefProc not in table)", "Message out of range", "Invalid (null) method", "Unknown message", "Manager call not supported", "Bad address", "Network operation in progress", "Network operation timed out", "Connection is busy", "Network attribute not supported", "Network error", "Address in use", "System out of memory", "Connection aborted", "Connection refused", "Not connected", "Already connected", "Connection closed", "Initialization error (interapplication manager)", "Bad occurrence", "Wait on unbound occurrence handler", "Occurrence queue overflow", "Datalog type conflict", "Unused", "Unrecognized type (interapplication manager)", "Memory corrupt", "Failed to make temporary DLL", "Old CIN version", "Drag socket not found", "Failed to load drop-object", "Failed to register OLE object", "Failed to release OLE object", "Format specifier type mismatch", "Unknown format specifier", "Too few format specifiers", "Too many format specifiers", "Scan failed", "Newer CIN version", "Error converting to variant", "Runtime menu error", "Password tampered", "Variant attribute not found", "Incompatible variant data type", "Event data is not available", "Event Store is not present", "Occurrence is not found", "Event Queue is not created", "Event info is not available", "Refnum passed is NULL", "Error retrieving Class GUID", "Error retrieving CoClass GUID", "Error retrieving TypeLib GUID.", "Bad built application magic bytes.", "Specific driver is different from the specific driver associated with the Logical Name.", "There is no session opened to the class driver.", "Max Error", "MAX - Error with config objects", "MAX - Error loading configuration", "MAX - Group not supported"]
        # "Do not delete, rename, or modify this frame.\n(this is used to capture unhandled states and typos)"
        # "Handle mistyped state name (developer tool)"
        n103 = Format Into String(format string="Software Exception: Unhandled State \"%s\"." ("message"), error in=w381, w376) -> (resulting string=w384:string, error out=w383:errorcluster)  [unwired: 1 in]
        n104 = call <vilib>:"Error Cluster From Error Code.vi"("show call chain? (False)"=TRUE, "error in (no error)"=w383, "error message (\"\")"=w384, "error code (0)"=w385) -> ("error out"=w382:errorcluster)  [unwired: 5 in]
        n105 = call <vilib>:"Add State(s) to Queue__JKI_lib_State_Machine.vi"("State(s) in (\"\")"=w380) -> ("States Out"=w379:string)  [unwired: 14 in]
      }
      frame "Error Handler" {
        # "Unhandled Error -- Display it"
        # "Handle any errors here.\nYou can also output any states to clean-up after errors occur"
        # "Clear error"
        n106 = call <vilib>:"General Error Handler.vi"("error in (no error)"=w388) -> ()  [unwired: 10 in, 5 out]
        n107 = call <vilib>:"Add State(s) to Queue__JKI_lib_State_Machine.vi"("State(s) in Front (\"\")"="/* Post Error States", "State(s) in (\"\")"=w392) -> ("States Out"=w391:string)  [unwired: 13 in]
      }
      frame "Critical Error" {
        w398 = 42 items=["No error", "Argument error", "Memory is full", "Out of zone", "End of file", "File already open", "Generic file I/O error", "File not found", "File permission error", "Disk is full", "Duplicate path", "Too many files open", "System feature not enabled", "Resource file not found", "Cannot add resource", "Resource not found", "Image not found", "Image memory error", "Pen does not exist", "Config type invalid", "Config token not found", "Config parse error", "Config memory error", "Bad external code format", "Bad external code offset", "External code not present", "Null window", "Destroy window error", "Null menu", "Print aborted", "Bad print record", "Print driver error", "Windows error during printing", "Memory error during printing", "Print dialog error", "Generic print error", "Invalid device refnum", "Device not found", "Device parameter error", "Device unit error", "Cannot open device", "Device call aborted", "Generic error", "Cancelled by user", "Object ID too low", "Object ID too high", "Object not in heap", "Unknown heap", "Unknown object (invalid DefProc)", "Unknown object (DefProc not in table)", "Message out of range", "Invalid (null) method", "Unknown message", "Manager call not supported", "Bad address", "Network operation in progress", "Network operation timed out", "Connection is busy", "Network attribute not supported", "Network error", "Address in use", "System out of memory", "Connection aborted", "Connection refused", "Not connected", "Already connected", "Connection closed", "Initialization error (interapplication manager)", "Bad occurrence", "Wait on unbound occurrence handler", "Occurrence queue overflow", "Datalog type conflict", "Unused", "Unrecognized type (interapplication manager)", "Memory corrupt", "Failed to make temporary DLL", "Old CIN version", "Drag socket not found", "Failed to load drop-object", "Failed to register OLE object", "Failed to release OLE object", "Format specifier type mismatch", "Unknown format specifier", "Too few format specifiers", "Too many format specifiers", "Scan failed", "Newer CIN version", "Error converting to variant", "Runtime menu error", "Password tampered", "Variant attribute not found", "Incompatible variant data type", "Event data is not available", "Event Store is not present", "Occurrence is not found", "Event Queue is not created", "Event info is not available", "Refnum passed is NULL", "Error retrieving Class GUID", "Error retrieving CoClass GUID", "Error retrieving TypeLib GUID.", "Bad built application magic bytes.", "Specific driver is different from the specific driver associated with the Logical Name.", "There is no session opened to the class driver.", "Max Error", "MAX - Error with config objects", "MAX - Error loading configuration", "MAX - Group not supported"]
        # "Handle critical error here.\nWhen any un-recoverable error occurs, CSM goes into this case."
        # "When Critical Error occurs, Stop the loop immediately. Do NOT change this unless you fully understand the impact."
        # "Handle mistyped state name (developer tool)"
        n108 = Format Into String(format string="Software Exception: Critical Error\"%s\"." ("message"), w394) -> (resulting string=w397:string, error out=w396:errorcluster)  [unwired: 2 in]
        n109 = call <vilib>:"Error Cluster From Error Code.vi"("show call chain? (False)"=TRUE, "error in (no error)"=w396, "error message (\"\")"=w397, "error code (0)"=w398) -> ()  [unwired: 5 in, 1 out]
        n110 = call <vilib>:"Add State(s) to Queue__JKI_lib_State_Machine.vi"("State(s) in (\"\")"=w401) -> ("States Out"=w400:string)  [unwired: 14 in]
      }
      frame "Target Timeout Error" {
        w413 = 42 items=["No error", "Argument error", "Memory is full", "Out of zone", "End of file", "File already open", "Generic file I/O error", "File not found", "File permission error", "Disk is full", "Duplicate path", "Too many files open", "System feature not enabled", "Resource file not found", "Cannot add resource", "Resource not found", "Image not found", "Image memory error", "Pen does not exist", "Config type invalid", "Config token not found", "Config parse error", "Config memory error", "Bad external code format", "Bad external code offset", "External code not present", "Null window", "Destroy window error", "Null menu", "Print aborted", "Bad print record", "Print driver error", "Windows error during printing", "Memory error during printing", "Print dialog error", "Generic print error", "Invalid device refnum", "Device not found", "Device parameter error", "Device unit error", "Cannot open device", "Device call aborted", "Generic error", "Cancelled by user", "Object ID too low", "Object ID too high", "Object not in heap", "Unknown heap", "Unknown object (invalid DefProc)", "Unknown object (DefProc not in table)", "Message out of range", "Invalid (null) method", "Unknown message", "Manager call not supported", "Bad address", "Network operation in progress", "Network operation timed out", "Connection is busy", "Network attribute not supported", "Network error", "Address in use", "System out of memory", "Connection aborted", "Connection refused", "Not connected", "Already connected", "Connection closed", "Initialization error (interapplication manager)", "Bad occurrence", "Wait on unbound occurrence handler", "Occurrence queue overflow", "Datalog type conflict", "Unused", "Unrecognized type (interapplication manager)", "Memory corrupt", "Failed to make temporary DLL", "Old CIN version", "Drag socket not found", "Failed to load drop-object", "Failed to register OLE object", "Failed to release OLE object", "Format specifier type mismatch", "Unknown format specifier", "Too few format specifiers", "Too many format specifiers", "Scan failed", "Newer CIN version", "Error converting to variant", "Runtime menu error", "Password tampered", "Variant attribute not found", "Incompatible variant data type", "Event data is not available", "Event Store is not present", "Occurrence is not found", "Event Queue is not created", "Event info is not available", "Refnum passed is NULL", "Error retrieving Class GUID", "Error retrieving CoClass GUID", "Error retrieving TypeLib GUID.", "Bad built application magic bytes.", "Specific driver is different from the specific driver associated with the Logical Name.", "There is no session opened to the class driver.", "Max Error", "MAX - Error with config objects", "MAX - Error loading configuration", "MAX - Group not supported"]
        # "Handle target timeout error here.\nWhen this CSM could not get the sync-call response in time, this CSM goes into this case."
        # "Handle mistyped state name (developer tool)"
        n111 = Format Into String(format string="Software Exception: Target could not finish the \"%s\" state in time." ("message"), error in=w409, w404) -> (resulting string=w412:string, error out=w411:errorcluster)  [unwired: 1 in]
        n112 = call <vilib>:"Error Cluster From Error Code.vi"("show call chain? (False)"=TRUE, "error in (no error)"=w411, "error message (\"\")"=w412, "error code (0)"=w413) -> ("error out"=w410:errorcluster)  [unwired: 5 in]
        n113 = call <vilib>:"Add State(s) to Queue__JKI_lib_State_Machine.vi"("State(s) in (\"\")"=w408) -> ("States Out"=w407:string)  [unwired: 14 in]
      }
      frame "Target Error" {
        w424 = 42 items=["No error", "Argument error", "Memory is full", "Out of zone", "End of file", "File already open", "Generic file I/O error", "File not found", "File permission error", "Disk is full", "Duplicate path", "Too many files open", "System feature not enabled", "Resource file not found", "Cannot add resource", "Resource not found", "Image not found", "Image memory error", "Pen does not exist", "Config type invalid", "Config token not found", "Config parse error", "Config memory error", "Bad external code format", "Bad external code offset", "External code not present", "Null window", "Destroy window error", "Null menu", "Print aborted", "Bad print record", "Print driver error", "Windows error during printing", "Memory error during printing", "Print dialog error", "Generic print error", "Invalid device refnum", "Device not found", "Device parameter error", "Device unit error", "Cannot open device", "Device call aborted", "Generic error", "Cancelled by user", "Object ID too low", "Object ID too high", "Object not in heap", "Unknown heap", "Unknown object (invalid DefProc)", "Unknown object (DefProc not in table)", "Message out of range", "Invalid (null) method", "Unknown message", "Manager call not supported", "Bad address", "Network operation in progress", "Network operation timed out", "Connection is busy", "Network attribute not supported", "Network error", "Address in use", "System out of memory", "Connection aborted", "Connection refused", "Not connected", "Already connected", "Connection closed", "Initialization error (interapplication manager)", "Bad occurrence", "Wait on unbound occurrence handler", "Occurrence queue overflow", "Datalog type conflict", "Unused", "Unrecognized type (interapplication manager)", "Memory corrupt", "Failed to make temporary DLL", "Old CIN version", "Drag socket not found", "Failed to load drop-object", "Failed to register OLE object", "Failed to release OLE object", "Format specifier type mismatch", "Unknown format specifier", "Too few format specifiers", "Too many format specifiers", "Scan failed", "Newer CIN version", "Error converting to variant", "Runtime menu error", "Password tampered", "Variant attribute not found", "Incompatible variant data type", "Event data is not available", "Event Store is not present", "Occurrence is not found", "Event Queue is not created", "Event info is not available", "Refnum passed is NULL", "Error retrieving Class GUID", "Error retrieving CoClass GUID", "Error retrieving TypeLib GUID.", "Bad built application magic bytes.", "Specific driver is different from the specific driver associated with the Logical Name.", "There is no session opened to the class driver.", "Max Error", "MAX - Error with config objects", "MAX - Error loading configuration", "MAX - Group not supported"]
        # "Handle target error here.\nWhen this CSM try to communicate with an un-existed CSM, this CSM goes into this case."
        # "Handle mistyped state name (developer tool)"
        n114 = Format Into String(format string="Software Exception: Target \"%s\" does not exists." ("message"), error in=w420, w415) -> (resulting string=w423:string, error out=w422:errorcluster)  [unwired: 1 in]
        n115 = call <vilib>:"Add State(s) to Queue__JKI_lib_State_Machine.vi"("State(s) in (\"\")"=w419) -> ("States Out"=w418:string)  [unwired: 14 in]
        n116 = call <vilib>:"Error Cluster From Error Code.vi"("show call chain? (False)"=TRUE, "error in (no error)"=w422, "error message (\"\")"=w423, "error code (0)"=w424) -> ("error out"=w421:errorcluster)  [unwired: 5 in]
      }
      frame "Async Response", "Response" {
        # "Handle Async-call Response (\"Async Response\" for ->)"
        # "Handle Sync-call Response (\"Response\" for @)"
        # "After Message is executed, CSM goes to this state for receive the response. \n    For Async Message(->), \"Async Response\" is used. This CSM will goes to \"Async Message Posted\" immediately and receive the \"Async Response\" after the callee finishes the message.\n    For Sync Message(@),  This CSM will wait until the message is done and immediately goes to \"Response\""
      }
      frame "Async Message Posted" {
        # "Handle post action for async message (->)."
        # "After Async Message is posted (->), CSM goes to this state for post-action. You can use Argument - State to tell which Async Message is called."
      }
      frame "Initialize Core Data" {
        # "Do not delete, rename, or modify this frame.\n(this is used to determine panel behavior on exit)"
        # "originally closed?"
        # "exe?"
        # "If panel starts closed or is an EXE, then close it when we exit"
        n117 = property class="VI"() -> ("FP.State"=w434:T1)  [unwired: 2 in, 2 out]
        n118 = property class="App"() -> ("App.Kind"=w440:T2)  [unwired: 2 in, 2 out]
        n119 = control-ref of="Current VI Reference"() -> (w435:refnum<vi>)
        n120 = Equal?(x=w434, y=T1."Closed" ("Front Panel Window:State")) -> (x = y?=w432:bool)
        n121 = Equal?(x=w440, y=T2."Run Time System" ("Application:Kind")) -> (x = y?=w438:bool)
        n122 = Or(x=w432, y=w438) -> (x .or. y?=w436:bool)
        n123 = Bundle By Name(cluster=w437, "Core.Current VI Reference"=w435, "Core.Close Panel on Exit?"=w436) -> (w442:T6)
        n124 = call <vilib>:"Add State(s) to Queue__JKI_lib_State_Machine.vi"("State(s) in (\"\")"=w444) -> ("States Out"=w443:string)  [unwired: 14 in]
      }
      frame "Exit" {
        # "Do not put any code in this frame.\n(No errors that occur here will be handled.)"
        n125 = call <vilib>:"Add State(s) to Queue__JKI_lib_State_Machine.vi"("State(s) in (\"\")"=w449) -> ("States Out"=w448:string)  [unwired: 14 in]
      }
      frame "---------- Data ----------" {
        # "Do not put any code in this frame.\n(It is a separator no-op. You can make a copy of this frame to create a new Data frame)"
        n126 = call <vilib>:"Add State(s) to Queue__JKI_lib_State_Machine.vi"("State(s) in (\"\")"=w453) -> ("States Out"=w452:string)  [unwired: 14 in]
      }
      frame "Data: Initialize" {
        w454 = T4 {"Current VI Reference"=refnum, "Close Panel on Exit?"=FALSE}  # Core
        w456 = TRUE  # Your Boolean data
        w455 = ""  # Your string data
        # "do not delete - used by framework"
        # "Expand Bundle to add new data elements to shift register data."
        # "Add new data here."
        # "Initialize the shift-register data, here.\n(data names are defined by what you wire into the bundle function)"
        n127 = Bundle("Core"=w454, "Your Boolean data"=w456, "Your string data"=w455) -> (w458:T6)  [unwired: 1 in]
        n128 = call <vilib>:"Add State(s) to Queue__JKI_lib_State_Machine.vi"("State(s) in (\"\")"=w460) -> ("States Out"=w459:string)  [unwired: 14 in]
      }
      frame "Data: Cleanup" {
        # "Cleanup any data and references, here.\n(this is called automatically, by the Macro: Exit)"
        n129 = Unbundle By Name(w461) -> ("Core.Current VI Reference"=w464:refnum<vi>)
        n130 = Close Reference(reference=w464, error in (no error)=w463) -> (error out=w462:errorcluster)
        n131 = call <vilib>:"Add State(s) to Queue__JKI_lib_State_Machine.vi"("State(s) in (\"\")"=w466) -> ("States Out"=w465:string)  [unwired: 14 in]
      }
      frame "---------- Macro ----------" {
        # "Do not put any code in this frame.\n(It is a separator no-op. You can make a copy of this frame to create a new Macro frame)"
        n132 = call <vilib>:"Add State(s) to Queue__JKI_lib_State_Machine.vi"("State(s) in (\"\")"=w470) -> ("States Out"=w469:string)  [unwired: 14 in]
      }
      frame "Macro: Initialize" {
        # "Initialization Macro\n(This is called once, when the VI starts)"
        n133 = call <vilib>:"Add State(s) to Queue__JKI_lib_State_Machine.vi"("State(s) in Front (\"\")"="Data: Initialize\nInitialize Core Data", "State(s) in (\"\")"=w475) -> ("States Out"=w474:string)  [unwired: 13 in]
      }
      frame "Macro: Exit" {
        # "Exit Macro\n(This is called once, when the VI exits)"
        n134 = call <vilib>:"Add State(s) to Queue__JKI_lib_State_Machine.vi"("State(s) in Front (\"\")"="Data: Cleanup\nExit", "State(s) in (\"\")"=w480) -> ("States Out"=w479:string)  [unwired: 13 in]
      }
      frame "---------- API ----------" {
        # "Do not put any code in this frame.\n(It is a separator no-op. This category is recommended to use for external API)"
      }
      frame "API: API1" {
        # "If you need to tell who triggered this state , use this string. If it's this case itself, this string is \"\"."
        # "Deal with the parameter if any"
        # "Connect this to return the response of your API"
        # "Copy/Rename this case for your own API"
      }
      frame "API: API2" {
        # "unpack HexStr  to Variant\nif complex parameter is needed."
        # "Copy/Rename this case for your own API"
        n135 = call "CSM - Convert HexStr to Data.vi"("HEX String"=w489) -> ()  [unwired: 7 in, 2 out]
        n136 = disable-structure shown="Enabled" {
          disable-tunnel: [w493 "API2 Response"] -> w488
          frame Disabled {
            # "pack variant to hexstr \nif complex response is needed."
            # "complex Response"
            n137 = call "CSM - Convert Data to HexStr.vi"() -> ("HEX String (0-9,A-F)"=w493:string)  [unwired: 9 in]
          }
          frame Enabled {
          }
        }
      }
      frame "---------- DoSth ----------" {
        # "Template Separator\n(You can make a copy of, or modify, this frame)"
        n138 = call <vilib>:"Add State(s) to Queue__JKI_lib_State_Machine.vi"("State(s) in (\"\")"=w498) -> ("States Out"=w497:string)  [unwired: 14 in]
      }
      frame "SM: Step2" {
        n139 = Wait (ms)(milliseconds to wait=u32 500) -> ()  [unwired: 1 out]
        n140 = call <vilib>:"Add State(s) to Queue__JKI_lib_State_Machine.vi"("State(s) in (\"\")"=w504) -> ("States Out"=w503:string)  [unwired: 14 in]
      }
      frame "SM: Step4" {
        n141 = Wait (ms)(milliseconds to wait=u32 500) -> ()  [unwired: 1 out]
        n142 = call <vilib>:"Add State(s) to Queue__JKI_lib_State_Machine.vi"("State(s) in (\"\")"=w510) -> ("States Out"=w509:string)  [unwired: 14 in]
      }
    }
  }
